vi "XL320_Initialize.vi"(7 "Timeout (30 msec)":u32=30, 8 "error in (no error)":errorcluster, 9 "Force Baud Rate (True)":bool, 10 "Baud rate (1,000,000 bps)":T1=3 items=["9600 bps", "57600 bps", "115200 bps", "1,000,000 bps"], 11 "VISA resource name":refnum<visa-resource-name>) -> (0 "error out":errorcluster, 3 "VISA resource name out":refnum<visa-resource-name>)   [LabVIEW 2017, in "Dynamixel XL320.lvlib"]
doc: "Establishes communication with the instrument and optionally performs an instrument identification query and/or an instrument reset. It also places the instrument in a default state needed for other instrument driver operations. Therefore, call this VI before calling other instrument driver VIs for this instrument. Generally, you need to call the Initialize VI only once at the beginning of an application."
uses:
  <instrlib>/Dynamixel XL320 (Drivers instrument)/Dynamixel XL320.lvlib
  <instrlib>/Dynamixel XL320 (Drivers instrument)/Public/Motor Operation/Low Level/XL320_Baud Setting.ctl
  <vilib>/Instr/_visa.llb/VISA Configure Serial Port (Instr).vi
panel:
  # "(c) 2011-2012  National Instruments.  ALL RIGHTS RESERVED."
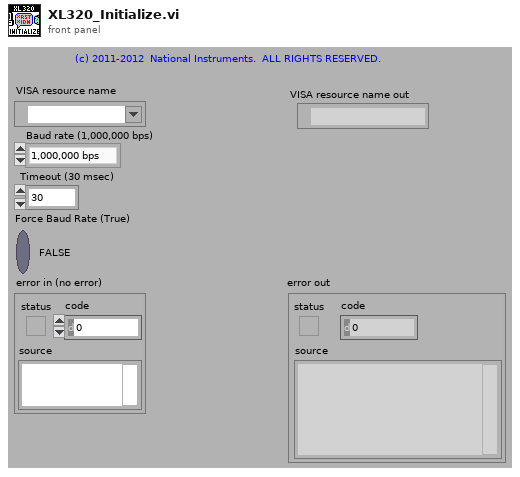
[diagram p1: front panel]
types:
  T1 = typedef "Dynamixel XL320.lvlib/XL320_Baud Setting.ctl" = u8
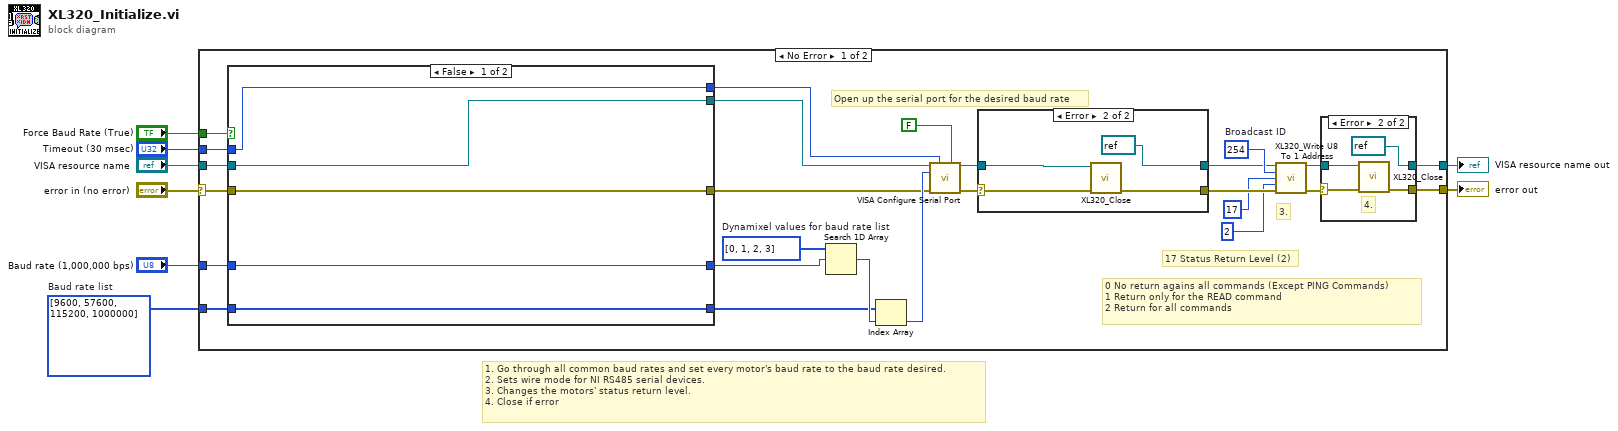
[diagram p0: block diagram]
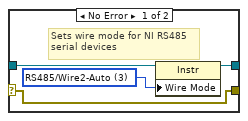
[diagram p2: hidden frame]
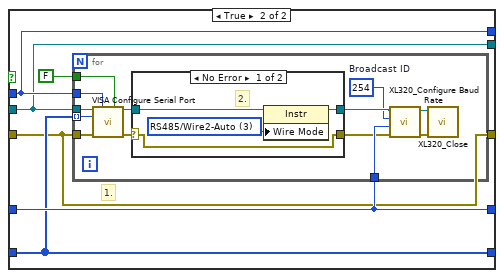
[diagram p3: hidden frame]
diagram:
  w3 = u32[] [9600, 57600, 115200, 1000000]  # Baud rate list
  # "1. Go through all common baud rates and set every motor's baud rate to the baud rate desired.\n2. Sets wire mode for NI RS485 serial devices.\n3. Changes the motors' status return level.\n4. Close if error"
  n1 = case shown="No Error" "error in (no error)" {
    selector: "error in (no error)" -> [w16 w80]
    tunnel: [w34 w79] -> w8
    tunnel: [w33 w80] -> w7
    tunnel: "VISA resource name" -> [w31 w79]
    tunnel: "Timeout (30 msec)" -> [w30 _]
    tunnel: "Baud rate (1,000,000 bps)" -> [w29 _]
    tunnel: "Force Baud Rate (True)" -> [w32 _]
    tunnel: w3 -> [w28 _]
    frame No Error {
      w26 = u8[] [0, 1, 2, 3]  # Dynamixel values for baud rate list
      w10 = u8 254  # Broadcast ID
      # "0 No return agains all commands (Except PING Commands)\n1 Return only for the READ command\n2 Return for all commands"
      # "17 Status Return Level (2)"
      # "Open up the serial port for the desired baud rate"
      # "3."
      n2 = case shown="False" w32 {
        tunnel: w31 -> [w43 w48]
        tunnel: w16 -> [w44 w49]
        tunnel: w30 -> [w45 w50]
        tunnel: w29 -> [w47 w52]
        tunnel: w28 -> [w46 w51]
        tunnel: [w47 w52] -> w21
        tunnel: [w46 w51] -> w20
        tunnel: [w45 w50] -> w19
        tunnel: [w44 w49] -> w18
        tunnel: [w43 w48] -> w17
        frame False {
        }
        frame True {
          # "1."
          n3 = for {
            tunnel: w48 -> [w66]
            tunnel: w49 -> [w65]
            tunnel: w50 -> [w64]
            tunnel: FALSE ("Enable Termination\nChar (T)") -> [w63]
            tunnel: w51 -> [w62] mode=indexing
            tunnel: w52 -> [w57]
            w58 = u8 254  # Broadcast ID
            n4 = call-poly "VISA Configure Serial Port"("VISA resource name"=w66, "timeout (10sec)"=w64, "Enable Termination\nChar (T)"=w63, "baud rate (9600)"=w62, "error in (no error)"=w65) -> ("VISA resource name out"=w61:refnum<visa-resource-name>, "error out"=w60:errorcluster)  [unwired: 9 in]
            n5 = case shown="No Error" w60 {
              selector: w60 -> [w67 w71]
              tunnel: w61 -> [w70 w72]
              tunnel: [w68 w72] -> w59
              tunnel: [w67 w71] -> w56
              frame No Error {
                w69 = i16 3 items=["Unknown"=-1, "RS485/Wire4"=0, "RS485/Wire2-EchoDTR"=1, "RS485/Wire2-CtrlDTR"=2, "RS485/Wire2-Auto"=3, "RS232/DTE"=128, "RS232/DCE"=129, "RS232/AUTO"=130] ("Serial Settings:Wire Mode")
                # "2."
                n6 = property class="Instr"(reference=w70, "Wire Mode"=w69) -> (reference out=w68:refnum<visa-resource-name>)  [unwired: 1 in, 1 out]
              }
              frame Error {
              }
            }
            n7 = call <instrlib>:"XL320_Configure Baud Rate.vi"("error in (no error)"=w56, "Baud rate (1,000,000 bps)"=w57, "Motor ID (0)"=w58, "VISA resource name"=w59) -> ("error out"=w54:errorcluster, "VISA resource name out"=w55:refnum<visa-resource-name>)  [unwired: 6 in]
            n8 = call <instrlib>:"XL320_Close.vi"("error in (no error)"=w54, "VISA resource name"=w55) -> ()  [unwired: 9 in, 1 out]
          }
        }
      }
      n9 = Search 1D Array(1D array=w26, element=w21) -> (index of element=w25:i32)  [unwired: 1 in]
      n10 = Index Array(array=w20, index=w25) -> (element=w24:u32)
      n11 = call-poly "VISA Configure Serial Port"("VISA resource name"=w17, "timeout (10sec)"=w19, "Enable Termination\nChar (T)"=FALSE ("Enable Termination\nChar (T)"), "baud rate (9600)"=w24, "error in (no error)"=w18) -> ("VISA resource name out"=w23:refnum<visa-resource-name>, "error out"=w22:errorcluster)  [unwired: 9 in]
      n12 = case shown="Error" w22 {
        selector: w22 -> [w38 w40]
        tunnel: w23 -> [w35 w41]
        tunnel: [w36 refnum<visa-resource-name> refnum ("VISA resource name out")] -> w9
        tunnel: [w38 w39] -> w13
        frame No Error {
          w37 = i16 3 items=["Unknown"=-1, "RS485/Wire4"=0, "RS485/Wire2-EchoDTR"=1, "RS485/Wire2-CtrlDTR"=2, "RS485/Wire2-Auto"=3, "RS232/DTE"=128, "RS232/DCE"=129, "RS232/AUTO"=130] ("Serial Settings:Wire Mode")
          # "Sets wire mode for NI RS485\nserial devices"
          n13 = property class="Instr"(reference=w35, "Wire Mode"=w37) -> (reference out=w36:refnum<visa-resource-name>)  [unwired: 1 in, 1 out]
        }
        frame Error {
          n14 = call <instrlib>:"XL320_Close.vi"("error in (no error)"=w40, "VISA resource name"=w41) -> ("error out"=w39:errorcluster)  [unwired: 9 in]
        }
      }
      n15 = call <instrlib>:"XL320_Write U8 To 1 Address.vi"("VISA resource name"=w9, "Motor ID (0)"=w10, "Address number (0)"=u16 17, "Parameter (0)"=u8 2, "error in (no error)"=w13) -> ("VISA resource name out"=w15:refnum<visa-resource-name>, "error out"=w14:errorcluster)  [unwired: 9 in]
      n16 = case shown="Error" w14 {
        selector: w14 -> [w74 w76]
        tunnel: [w73 refnum<visa-resource-name> refnum ("VISA resource name out")] -> w34
        tunnel: [w74 w75] -> w33
        tunnel: w15 -> [w73 w77]
        frame No Error {
        }
        frame Error {
          # "4."
          n17 = call <instrlib>:"XL320_Close.vi"("error in (no error)"=w76, "VISA resource name"=w77) -> ("error out"=w75:errorcluster)  [unwired: 9 in]
        }
      }
    }
    frame Error {
    }
  }
  "VISA resource name out" <- w8
  "error out" <- w7
